vi "RT Motors Module.vi"(1 "Speed":T1, 3 "Error In":errorcluster, 4 "All":T2, 5 "FPGA VI Reference In":refnum<k20>) -> (0 "Error Out":errorcluster, 2 "FPGA VI Reference Out":refnum<k20>)   [LabVIEW 2015]
uses:
  <vilib>/Utility/error.llb/Error Cluster From Error Code.vi
  <vilib>/rvi/errors/niLvFpgaAdjustHostInterfaceError.vi
  <vilib>/rvi/interface/nirviReadWriteControl/nirviReadWriteControl.xnode
  NiFpgaLv.dll
  <vilib>/rvi/interface/Simulation/niFpgaSimulationCallBeginRW.vi
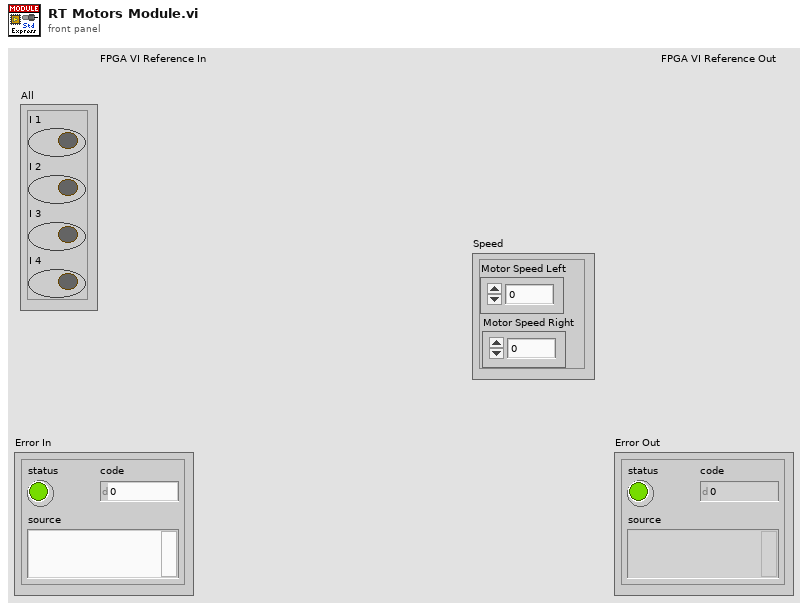
[diagram p1: front panel]
types:
  T1 = cluster{"Motor Speed Left":i16, "Motor Speed Right":i16}
  T2 = cluster{"I 1":bool, "I 2":bool, "I 3":bool, "I 4":bool}
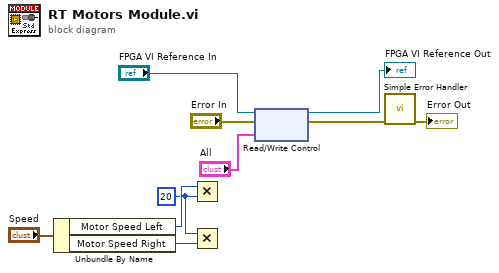
[diagram p0: block diagram]
diagram:
  w2 = i16 20 ("y")
  n1 = Unbundle By Name("Speed") -> ("Motor Speed Left"=w3:i16, "Motor Speed Right"=w1:i16)
  n2 = Multiply(x=w3, y=w2) -> ()  [unwired: 1 out]
  n3 = Multiply(x=w2, y=w1) -> ()  [unwired: 1 out]
  n4 = xnode "Read/Write Control"("FPGA VI Reference In"="FPGA VI Reference In", "error in"="Error In", "Mot F"="All") -> ("FPGA VI Reference Out"=→"FPGA VI Reference Out":refnum<k20>, "error out"=w7:errorcluster)
  n5 = call <vilib>:"Simple Error Handler.vi"("error in (no error)"=w7) -> ("error out"=→"Error Out":errorcluster)  [unwired: 4 in, 4 out]
